vi "PathPlanner_PathSegment_New.vi"(5 "P1":T5 {"Y" format="%14.3f"; "X" format="%14.3f"}, 6 "EndSegment":bool, 7 "P2":T5 {"Y" format="%14.3f"; "X" format="%14.3f"}, 8 "ConstraintZones":T1[](array[typedef]), 9 "TargetHolonomicRotations":T3[](array[typedef]) {"rotation"."SIN" format="%13.4f"; "rotation"."COS" format="%13.4f"; "rotation"."VALUE" format="%13.4f"}, 10 "P4":T5 {"Y" format="%14.3f"; "X" format="%14.3f"}, 11 "P3":T5 {"Y" format="%14.3f"; "X" format="%14.3f"}) -> (3 "Segment":T6 {"SegmentPoints"."RotationTarget"."rotation"."SIN" format="%13.4f"; "SegmentPoints"."RotationTarget"."rotation"."COS" format="%13.4f"; "SegmentPoints"."RotationTarget"."rotation"."VALUE" format="%13.4f"; "SegmentPoints"."Position"."Y" format="%14.3f"; "SegmentPoints"."Position"."X" format="%14.3f"})   [LabVIEW 2019, in "PathPlanner24.lvlib"]
doc: "Generate a new path segment\n\nInputs: \n - p1 - translation2d - Start anchor point\n - p2 - translation2d - Start next control\n - p3 - translation2d - End prev control\n - p4 - translation2d - End anchor point\n - targetHolonomicRotations - array Rotation targets for within this segment (Optional. Default: empty)\n - constraintZones - array - Constraint zones for within this segment (Optional. Default: empty)\n - endSegment - boolean - Is this the last segment in the path\n\nOutputs:\n - Segment - cluster - Data defining path segment"
uses:
  PathPlanner24.lvlib
  TypeDef/PathPlannerPathConstraints.ctl
  <vilib>/Rock Robotics/WPI/ThirdParty/JAS_Junk/TrajLib/TypeDef/TRANSLATION2D.ctl
  <vilib>/Rock Robotics/WPI/ThirdParty/JAS_Junk/TrajLib/Trajectory_Library.lvlib
  <vilib>/Rock Robotics/WPI/ThirdParty/JAS_Junk/TrajLib/TypeDef/ROTATION2D.ctl
  TypeDef/PathPlannerPathPoint.ctl
  TypeDef/PathPlannerPathSegment.ctl
  TypeDef/PathPlannerRotationTarget.ctl
  TypeDef/PathPlannerConstraintsZone.ctl
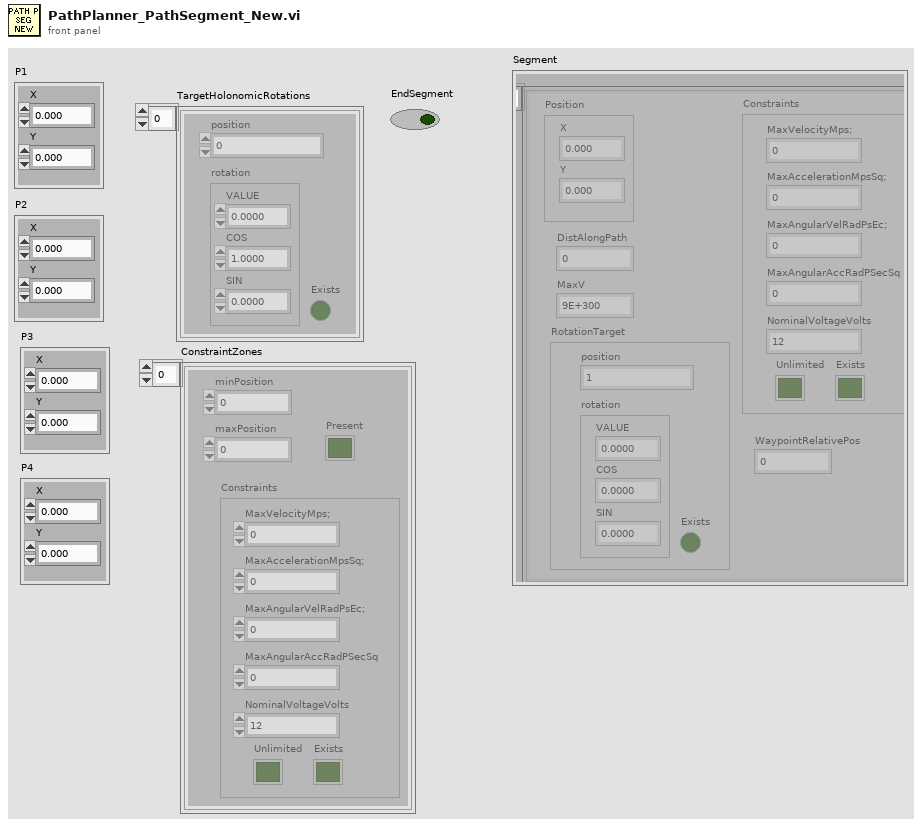
[diagram p1: front panel]
types:
  T1 = typedef "PathPlanner24.lvlib/PathPlannerConstraintsZone.ctl" = cluster{"minPosition":dbl, "maxPosition":dbl, "Constraints":T2, "Present":bool}
  T2 = typedef "PathPlanner24.lvlib/PathPlannerPathConstraints.ctl" = cluster{"MaxVelocityMps;":dbl, "MaxAccelerationMpsSq;":dbl, "MaxAngularVelRadPsEc;":dbl, "MaxAngularAccRadPSecSq":dbl, "Exists":bool, "Unlimited":bool, "NominalVoltageVolts":dbl}
  T3 = typedef "PathPlanner24.lvlib/PathPlannerRotationTarget.ctl" = cluster{"rotation":T4, "position":dbl, "Exists":bool}
  T4 = typedef "Trajectory_Library.lvlib/ROTATION2D.ctl" = cluster{"VALUE":dbl, "COS":dbl, "SIN":dbl}
  T5 = typedef "Trajectory_Library.lvlib/TRANSLATION2D.ctl" = cluster{"X":dbl, "Y":dbl}
  T6 = typedef "PathPlanner24.lvlib/PathPlannerPathSegment.ctl" = cluster{"SegmentPoints":T7[]}
  T7 = typedef "PathPlanner24.lvlib/PathPlannerPathPoint.ctl" = cluster{"Position":T5, "DistAlongPath":dbl, "MaxV":dbl, "Constraints":T2, "RotationTarget":T3, "WaypointRelativePos":dbl}
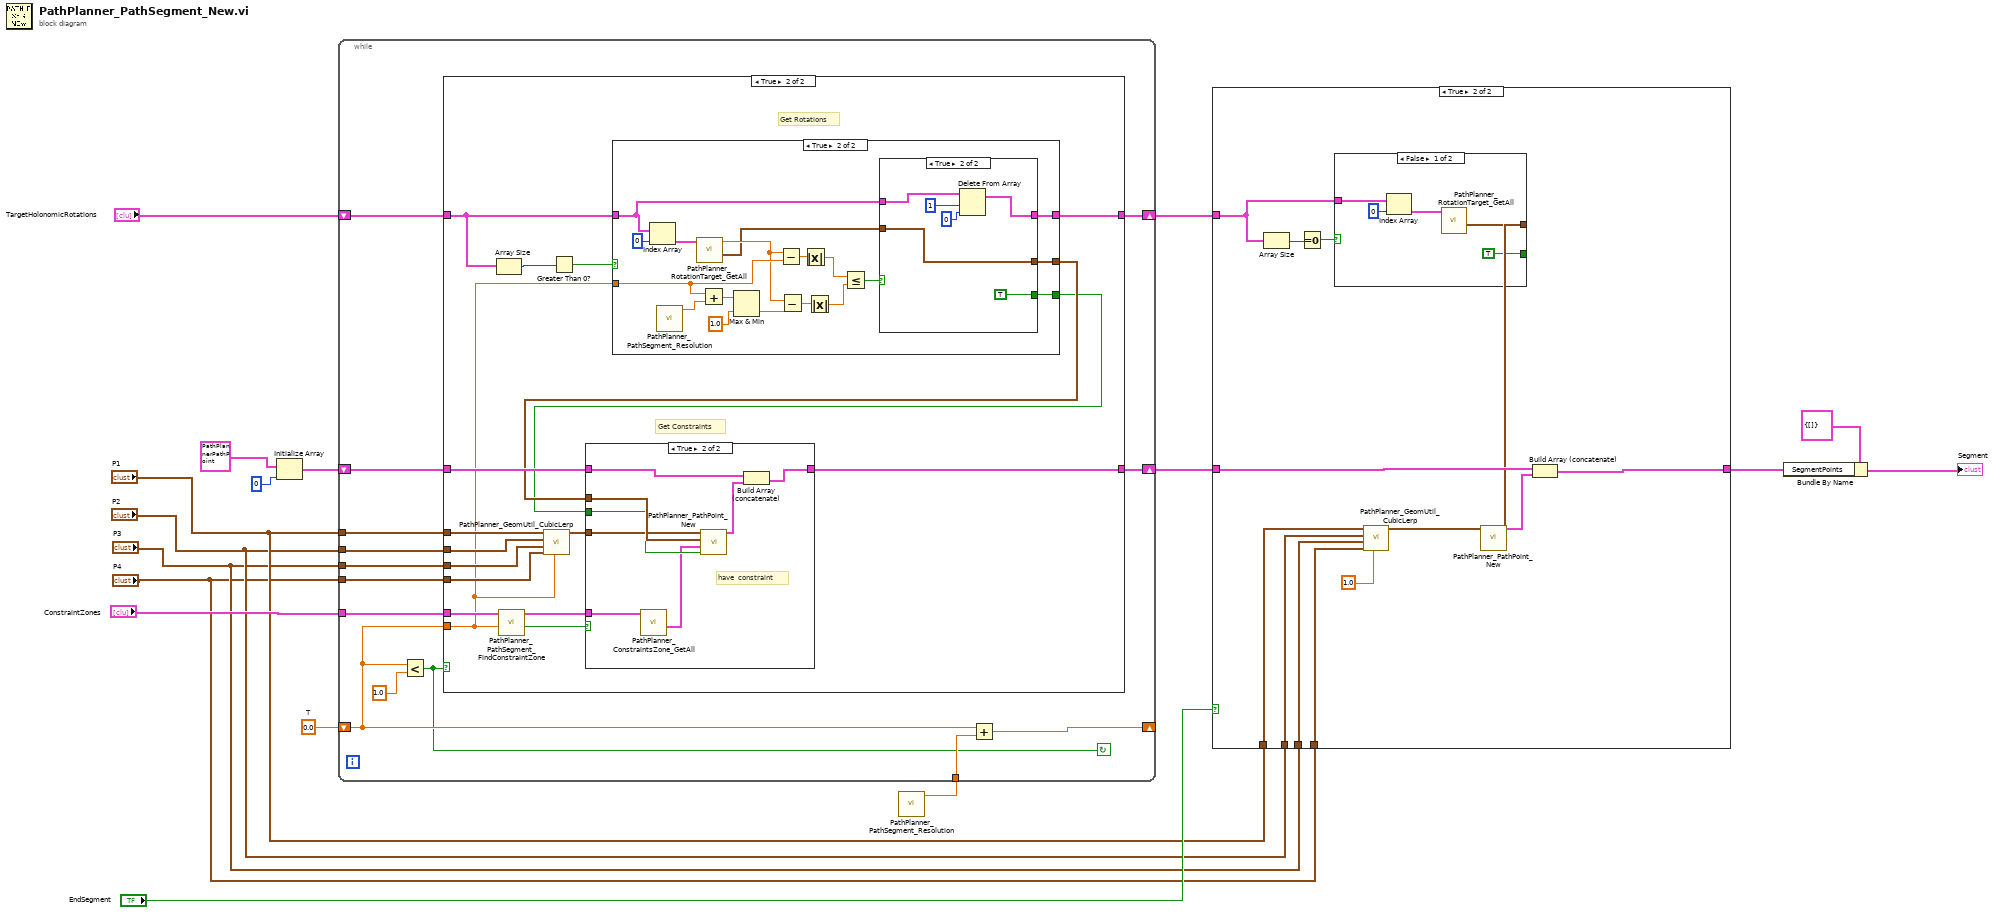
[diagram p0: block diagram]
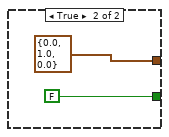
[diagram p3: hidden frame]
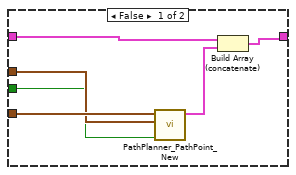
[diagram p5: hidden frame]
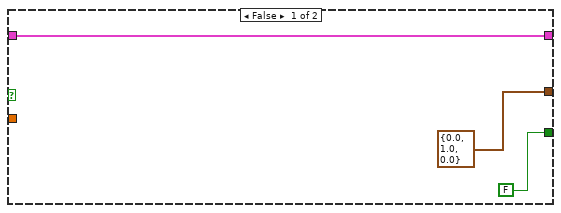
[diagram p6: hidden frame]
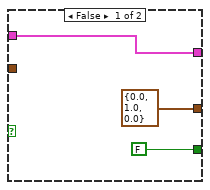
[diagram p7: hidden frame]
diagram:
  w15 = 0.0  # T
  n1 = Initialize Array(T7 {"Position"={"X"=0.0, "Y"=0.0}, "DistAlongPath"=0.0, "MaxV"=9e+300, "Constraints"={"MaxVelocityMps;"=0.0, "MaxAccelerationMpsSq;"=0.0, "MaxAngularVelRadPsEc;"=0.0, "MaxAngularAccRadPSecSq"=0.0, "Exists"=FALSE, "Unlimited"=FALSE, "NominalVoltageVolts"=12.0}, "RotationTarget"={"rotation"={"VALUE"=0.0, "COS"=0.0, "SIN"=0.0}, "position"=1.0, "Exists"=FALSE}, "WaypointRelativePos"=0.0} ("PathPlannerPoint"), 0 ("dimension size")) -> (w11:T7[])
  n2 = call "PathPlanner_PathSegment_Resolution.vi"() -> ("Resolution"=w14:dbl)  [unwired: 11 in]
  n3 = while {
    shift-right: [w19] -> _
    shift-left: w15 -> [w21]
    tunnel: w14 -> [w31]
    tunnel: "ConstraintZones" -> [w28]
    shift-right: [w29] -> w5
    shift-left: "TargetHolonomicRotations" -> [w30]
    shift-right: [w22] -> w9
    shift-left: w11 -> [w27]
    tunnel: "P1" -> [w26]
    tunnel: "P2" -> [w25]
    tunnel: "P3" -> [w24]
    tunnel: "P4" -> [w23]
    stop <- w18 continue-if-true
    n4 = Less?(x=w21, y=1.0) -> (x < y?=w18:bool)
    n5 = case shown="True" w18 {
      tunnel: w30 -> [w33 w50]
      tunnel: [w33 w49] -> w29
      tunnel: w28 -> [_ w48]
      tunnel: w27 -> [w32 w47]
      tunnel: w26 -> [_ w46]
      tunnel: w25 -> [_ w45]
      tunnel: w24 -> [_ w44]
      tunnel: w23 -> [_ w43]
      tunnel: [w32 w42] -> w22
      tunnel: w21 -> [_ w34]
      frame False {
      }
      frame True {
        # "Get Constraints"
        # "Get Rotations"
        n6 = Array Size(array=w50) -> (size(s)=w36:i32)
        n7 = call "PathPlanner_PathSegment_FindConstraintZone.vi"("T"=w34, "Zones"=w48) -> ("IsPresent"=w37:bool, "Returned Zone"=w39:T1)  [unwired: 8 in]
        n8 = call "PathPlanner_GeomUtil_CubicLerp.vi"("T"=w34, "D"=w43, "C"=w44, "B"=w45, "A"=w46) -> ("Lerp"=w38:T5)  [unwired: 6 in]
        n9 = Greater Than 0?(x=w36) -> (x > 0?=w35:bool)
        n10 = case shown="True" w35 {
          tunnel: w50 -> [w67 w70]
          tunnel: [w67 w69] -> w49
          tunnel: w34 -> [_ w81]
          tunnel: [T4 {"VALUE"=0.0, "COS"=1.0, "SIN"=0.0} ("ROTATION") w72] -> w41
          tunnel: [FALSE w68] -> w40
          frame False {
          }
          frame True {
            n11 = Index Array(array=w70, index=0) -> (element=w84:T3)
            n12 = call "PathPlanner_PathSegment_Resolution.vi"() -> ("Resolution"=w82:dbl)  [unwired: 11 in]
            n13 = call "PathPlanner_RotationTarget_GetAll.vi"("RotationTarget"=w84) -> ("rotation"=w71:T4, "position"=w77:dbl)  [unwired: 8 in, 1 out]
            n14 = Add(x=w81, y=w82) -> (x+y=w80:dbl)
            n15 = Max & Min(x=w80, y=1.0) -> (min(x,y)=w78:dbl)  [unwired: 1 out]
            n16 = Subtract(x=w77, y=w81) -> (x-y=w83:dbl)
            n17 = Subtract(x=w77, y=w78) -> (x-y=w76:dbl)
            n18 = Absolute Value(x=w83) -> (abs(x)=w74:dbl)
            n19 = Absolute Value(x=w76) -> (abs(x)=w75:dbl)
            n20 = Less Or Equal?(x=w74, y=w75) -> (x <= y?=w73:bool)
            n21 = case shown="True" w73 {
              tunnel: [T4 {"VALUE"=0.0, "COS"=1.0, "SIN"=0.0} ("ROTATION") w94] -> w72
              tunnel: w71 -> [_ w94]
              tunnel: w70 -> [w87 w93]
              tunnel: [w87 w90] -> w69
              tunnel: [FALSE TRUE] -> w68
              frame False {
              }
              frame True {
                n22 = Delete From Array(array=w93, length=1, index=0) -> (array with subset deleted=w90:T3[])  [unwired: 1 out]
              }
            }
          }
        }
        n23 = case shown="True" w37 {
          tunnel: w47 -> [w55 w64]
          tunnel: [w54 w63] -> w42
          tunnel: w41 -> [w52 w62]
          tunnel: w40 -> [w51 w61]
          tunnel: w39 -> [_ w60]
          tunnel: w38 -> [w53 w58]
          frame False {
            n24 = call "PathPlanner_PathPoint_New.vi"(8:w51, "RotationTarget"=w52, "Position"=w53) -> ("PathPlannerPoint"=w56:T7)  [unwired: 8 in]
            n25 = Build Array (concatenate)(w55, w56) -> (w54:T7[])
          }
          frame True {
            # "have  constraint"
            n26 = call "PathPlanner_ConstraintsZone_GetAll.vi"("ConstraintsZone"=w60) -> ("Constraints"=w57:T2)  [unwired: 8 in, 2 out]
            n27 = call "PathPlanner_PathPoint_New.vi"(8:w61, "Constraints"=w57, "RotationTarget"=w62, "Position"=w58) -> ("PathPlannerPoint"=w59:T7)  [unwired: 7 in]
            n28 = Build Array (concatenate)(w64, w59) -> (w63:T7[])
          }
        }
      }
    }
    n29 = Add(x=w21, y=w31) -> (x+y=w19:dbl)
  }
  n30 = case shown="True" "EndSegment" {
    tunnel: w9 -> [w95 w101]
    tunnel: [w95 w100] -> w6
    tunnel: w5 -> [_ w107]
    tunnel: "P1" -> [_ w106]
    tunnel: "P2" -> [_ w99]
    tunnel: "P3" -> [_ w105]
    tunnel: "P4" -> [_ w104]
    frame False {
    }
    frame True {
      n31 = Array Size(array=w107) -> (size(s)=w109:i32)
      n32 = Equal To 0?(x=w109) -> (x = 0?=w108:bool)
      n33 = case shown="False" w108 {
        tunnel: w107 -> [w113 _]
        tunnel: [w111 T4 {"VALUE"=0.0, "COS"=1.0, "SIN"=0.0} ("ROTATION")] -> w97
        tunnel: [TRUE FALSE] -> w96
        frame False {
          n34 = Index Array(array=w113, index=0) -> (element=w112:T3)
          n35 = call "PathPlanner_RotationTarget_GetAll.vi"("RotationTarget"=w112) -> ("rotation"=w111:T4)  [unwired: 8 in, 2 out]
        }
        frame True {
        }
      }
      n36 = call "PathPlanner_GeomUtil_CubicLerp.vi"("T"=1.0, "D"=w104, "C"=w105, "B"=w99, "A"=w106) -> ("Lerp"=w98:T5)  [unwired: 6 in]
      n37 = call "PathPlanner_PathPoint_New.vi"(8:w96, "RotationTarget"=w97, "Position"=w98) -> ("PathPlannerPoint"=w102:T7)  [unwired: 8 in]
      n38 = Build Array (concatenate)(w101, w102) -> (w100:T7[])
    }
  }
  n39 = Bundle By Name(cluster=T6 {"SegmentPoints"=[]} ("Segment"), "SegmentPoints"=w6) -> (→"Segment":T6)
